vi "Sensor Hysteresis (SubVI).vi"(9 "Hysteresis":dbl, 10 "Input":dbl, 11 "Threshold":dbl) -> (3 "Above Threshold":bool)   [LabVIEW 2020]
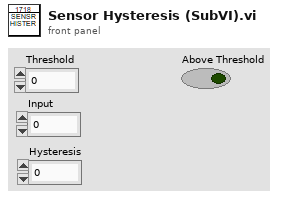
[diagram p1: front panel]
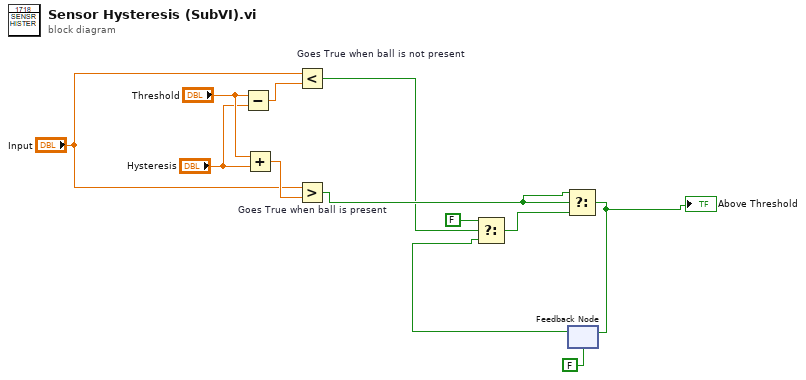
[diagram p0: block diagram]
diagram:
  n1 = Subtract(x="Threshold", y="Hysteresis") -> (x-y=w11:dbl)
  n2 = Add(x="Threshold", y="Hysteresis") -> (x+y=w12:dbl)
  n3 = Less? "Goes True when ball is not present"(x="Input", y=w11) -> (x < y?=w2:bool)
  n4 = Greater? "Goes True when ball is present"(x="Input", y=w12) -> (0:w6:bool)
  n5 = feedback #1(FALSE) -> (w4:bool)
  n6 = Select(t=FALSE, s=w2, f=w4) -> (s? t:f=w3:bool)
  n7 = Select(t=w6, s=w6, f=w3) -> (s? t:f=w5:bool)
  "Above Threshold" <- w5
  n8 = feedback-in #1(w5) -> ()
